vi "MPB Signal Reads.vi"() -> (3 "RX Signals":string[](array[string])=["AEthernet.Powertrain.TCU.RX_PDUs.MPB_STS_1.IMPB_CntctSts1", "AEthernet.Powertrain.TCU.RX_PDUs.MPB_STS_1.IMPB_CntctSts2", "AEthernet.Powertrain.TCU.RX_PDUs.MPB_STS_1.IMPB_CntctSts3", "AEthernet.Powertrain.TCU.RX_PDUs.MPB_STS_1.IMPB_CntctSts4", "AEthernet.Powertrain.TCU.RX_PDUs.MPB_STS_1.IMPB_CntctSts5", "AEthernet.Powertrain.TCU.RX_PDUs.MPB_STS_1.IMPB_CntctSts6", "AEthernet.Powertrain.TCU.RX_PDUs.MPB_STS_1.IMPB_CntctSts7", "AEthernet.Powertrain.TCU.RX_PDUs.MPB_STS_1.IMPB_RlySts1", "AEthernet.Powertrain.TCU.RX_PDUs.MPB_STS_1.IMPB_RlySts2", "AEthernet.Powertrain.TCU.RX_PDUs.MPB_STS_1.IMPB_BattCurrDAB1", "AEthernet.Powertrain.TCU.RX_PDUs.MPB_STS_1.IMPB_BattCurrDAB2", "AEthernet.Powertrain.TCU.RX_PDUs.MPB_STS_1.IMPB_BattVoltgHiRes", "AEthernet.Powertrain.TCU.RX_PDUs.MPB_STS_1.IMPB_DCbusVoltg", "AEthernet.Powertrain.TCU.RX_PDUs.MPB_STS_1.IMPB_BattPortPower", "AEthernet.Powertrain.TCU.RX_PDUs.MPB_STS_1.IMPB_InletDCportVoltgHiRes", "AEthernet.Powertrain.TCU.RX_PDUs.MPB_INLET_1.IMPB_DCbusVoltgLowrHalf", "AEthernet.Powertrain.TCU.RX_PDUs.MPB_STS_1.IMPB_BattPortVoltgLowRes", "AEthernet.Powertrain.TCU.RX_PDUs.MPB_HAPS.IMPB_HAPSVoltgIn", "AEthernet.Powertrain.TCU.RX_PDUs.MPB_HwFlt.IMPB_HwFltCode", "AEthernet.Powertrain.TCU.RX_PDUs.MPB_STS_1.IMPB_BattPortNegFuseLowRes", "AEthernet.Powertrain.TCU.RX_PDUs.MPB_STS_1.IMPB_BattPortPosFuseLowRes", "AEthernet.Powertrain.TCU.RX_PDUs.MPB_HwFlt.IMPB_HwFltFlag", "AEthernet.Powertrain.TCU.RX_PDUs.MPB_ACCURR.IMPB_ACCurr1", "AEthernet.Powertrain.TCU.RX_PDUs.MPB_ACCURR.IMPB_ACCurr2", "AEthernet.Powertrain.TCU.RX_PDUs.MPB_ACCURR.IMPB_ACCurr3", "AEthernet.Powertrain.TCU.RX_PDUs.MPB_ACCURR.IMPB_ACCurr4", "AEthernet.Powertrain.TCU.RX_PDUs.MPB_HAPS.IMPB_HAPSCurr", "AEthernet.Powertrain.TCU.RX_PDUs.MPB_HAPS.IMPB_HAPSVoltgOut", "AEthernet.Powertrain.TCU.RX_PDUs.MPB_HAPS.IMPB_HAPSFltFlag", "AEthernet.Powertrain.TCU.RX_PDUs.MPB_HAPS.IMPB_HAPSFltCode"])   [LabVIEW 2020]
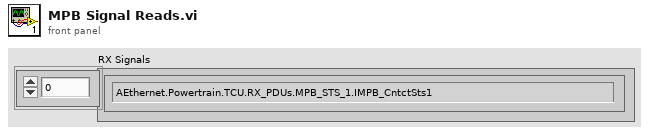
[diagram p1: front panel]
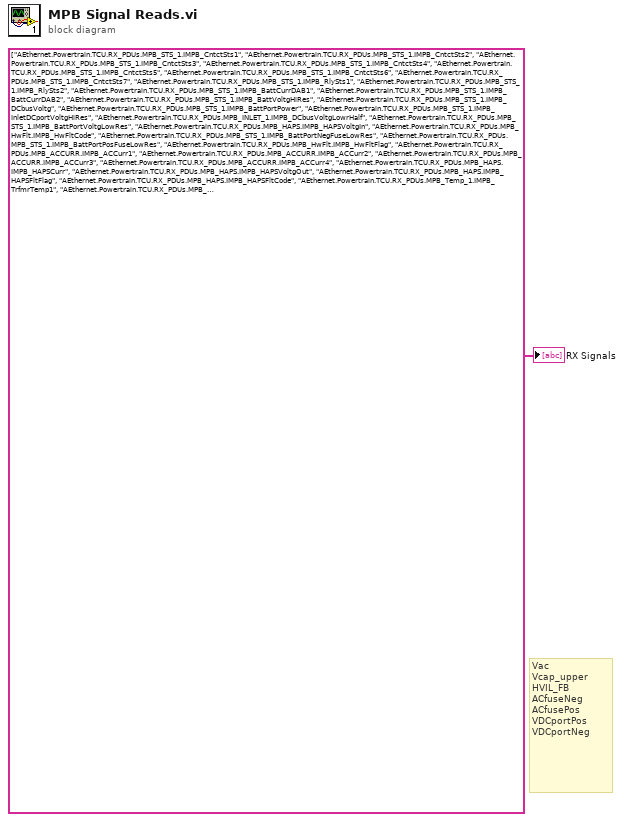
[diagram p0: block diagram]
diagram:
  # "Vac\nVcap_upper\nHVIL_FB\nACfuseNeg\nACfusePos\nVDCportPos\nVDCportNeg"
  "RX Signals" <- string[] ["AEthernet.Powertrain.TCU.RX_PDUs.MPB_STS_1.IMPB_CntctSts1", "AEthernet.Powertrain.TCU.RX_PDUs.MPB_STS_1.IMPB_CntctSts2", "AEthernet.Powertrain.TCU.RX_PDUs.MPB_STS_1.IMPB_CntctSts3", "AEthernet.Powertrain.TCU.RX_PDUs.MPB_STS_1.IMPB_CntctSts4", "AEthernet.Powertrain.TCU.RX_PDUs.MPB_STS_1.IMPB_CntctSts5", "AEthernet.Powertrain.TCU.RX_PDUs.MPB_STS_1.IMPB_CntctSts6", "AEthernet.Powertrain.TCU.RX_PDUs.MPB_STS_1.IMPB_CntctSts7", "AEthernet.Powertrain.TCU.RX_PDUs.MPB_STS_1.IMPB_RlySts1", "AEthernet.Powertrain.TCU.RX_PDUs.MPB_STS_1.IMPB_RlySts2", "AEthernet.Powertrain.TCU.RX_PDUs.MPB_STS_1.IMPB_BattCurrDAB1", "AEthernet.Powertrain.TCU.RX_PDUs.MPB_STS_1.IMPB_BattCurrDAB2", "AEthernet.Powertrain.TCU.RX_PDUs.MPB_STS_1.IMPB_BattVoltgHiRes", "AEthernet.Powertrain.TCU.RX_PDUs.MPB_STS_1.IMPB_DCbusVoltg", "AEthernet.Powertrain.TCU.RX_PDUs.MPB_STS_1.IMPB_BattPortPower", "AEthernet.Powertrain.TCU.RX_PDUs.MPB_STS_1.IMPB_InletDCportVoltgHiRes", "AEthernet.Powertrain.TCU.RX_PDUs.MPB_INLET_1.IMPB_DCbusVoltgLowrHalf", "AEthernet.Powertrain.TCU.RX_PDUs.MPB_STS_1.IMPB_BattPortVoltgLowRes", "AEthernet.Powertrain.TCU.RX_PDUs.MPB_HAPS.IMPB_HAPSVoltgIn", "AEthernet.Powertrain.TCU.RX_PDUs.MPB_HwFlt.IMPB_HwFltCode", "AEthernet.Powertrain.TCU.RX_PDUs.MPB_STS_1.IMPB_BattPortNegFuseLowRes", "AEthernet.Powertrain.TCU.RX_PDUs.MPB_STS_1.IMPB_BattPortPosFuseLowRes", "AEthernet.Powertrain.TCU.RX_PDUs.MPB_HwFlt.IMPB_HwFltFlag", "AEthernet.Powertrain.TCU.RX_PDUs.MPB_ACCURR.IMPB_ACCurr1", "AEthernet.Powertrain.TCU.RX_PDUs.MPB_ACCURR.IMPB_ACCurr2", "AEthernet.Powertrain.TCU.RX_PDUs.MPB_ACCURR.IMPB_ACCurr3", "AEthernet.Powertrain.TCU.RX_PDUs.MPB_ACCURR.IMPB_ACCurr4", "AEthernet.Powertrain.TCU.RX_PDUs.MPB_HAPS.IMPB_HAPSCurr", "AEthernet.Powertrain.TCU.RX_PDUs.MPB_HAPS.IMPB_HAPSVoltgOut", "AEthernet.Powertrain.TCU.RX_PDUs.MPB_HAPS.IMPB_HAPSFltFlag", "AEthernet.Powertrain.TCU.RX_PDUs.MPB_HAPS.IMPB_HAPSFltCode", "AEthernet.Powertrain.TCU.RX_PDUs.MPB_Temp_1.IMPB_TrfmrTemp1", "AEthernet.Powertrain.TCU.RX_PDUs.MPB_Temp_1.IMPB_TrfmrTemp2", "AEthernet.Powertrain.TCU.RX_PDUs.MPB_STS_1.IMPB_InletACportVoltgHiRes", "AEthernet.Powertrain.TCU.RX_PDUs.MPB_INLET_1.IMPB_DCbusVoltgUpprHalf", "AEthernet.Powertrain.TCU.RX_PDUs.MPB_STS_1.IMPB_HeatgActv", "AEthernet.Powertrain.TCU.RX_PDUs.MPB_INLET_2.IMPB_InletACportEgy", "AEthernet.Powertrain.TCU.RX_PDUs.MPB_STS_1.IMPB_InletACportFuseLowRes", "AEthernet.Powertrain.TCU.RX_PDUs.MPB_STS_1.IMPB_InletDCportPosLowRes", "AEthernet.Powertrain.TCU.RX_PDUs.MPB_STS_1.IMPB_InletDCportNegLowRes"]
